vi "Destroy User Events.vi"(11 "UI Template in":refnum<class "UI_Top.lvclass">) -> (3 "UI Template out":refnum<class "UI_Top.lvclass">)   [LabVIEW 2021, in "UI_Top.lvclass"]
uses:
  UI_Top.lvclass
  UI_Top.lvclass/UI_Top.ctl
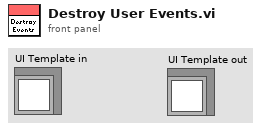
[diagram p1: front panel]
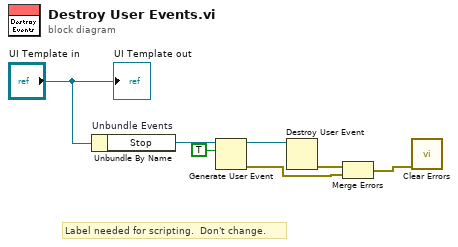
[diagram p0: block diagram]
diagram:
  # "Label needed for scripting.  Don't change."
  n1 = Unbundle By Name "Unbundle Events"("UI Template in") -> ("Stop"=w5:refnum<user-event>)
  n2 = Generate User Event(user event=w5, event data cluster=TRUE ("event data")) -> (user event out=w6:refnum<user-event>, error out=w1:errorcluster)  [unwired: 2 in]
  n3 = Destroy User Event(user event=w6) -> (error out=w3:errorcluster)  [unwired: 1 in]
  n4 = Merge Errors(w3, w1) -> (w2:errorcluster)
  n5 = call <vilib>:"Clear Errors.vi"("error in (no error)"=w2) -> ()  [unwired: 5 in, 2 out]
  "UI Template out" <- "UI Template in"
